vi "Identify Head vs Tail in Difference Image.vi"(8 "significance level":dbl=0.01, 9 "History Length \nfor Head v Tail Determination":i32=100, 10 "Reset?":bool, 11 "Diff Image In":T1) -> (2 "Significant?":bool, 3 "Facing Left?":bool)   [LabVIEW 2011]
uses:
  <vilib>/vision/Image Controls.llb/IMAQ Image.ctl
  <vilib>/Analysis/3filter.llb/Filter Passband Type.ctl
  <vilib>/gmath/statdist.llb/Wilcoxon Signed-Rank Test (mean).vi
  <vilib>/ptbypt/NI_PtbyPt.lvlib
  <vilib>/gmath/NI_Gmath.lvlib
  <vilib>/Analysis/NI_AALBase.lvlib
panel:
  out "Left/Right Diff Sum":i16(graph)
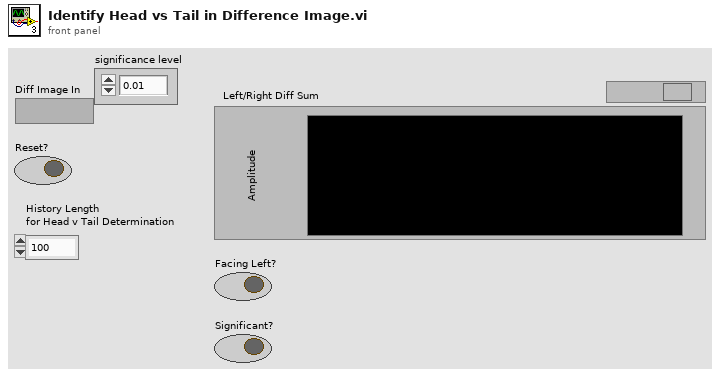
[diagram p1: front panel]
types:
  T1 = typedef "IMAQ Image.ctl" = refnum<image>
  T2 = typedef "NI_AALBase.lvlib/Filter Passband Type.ctl" = enum32{"Lowpass", "Highpass", "Bandpass", "Bandstop"}
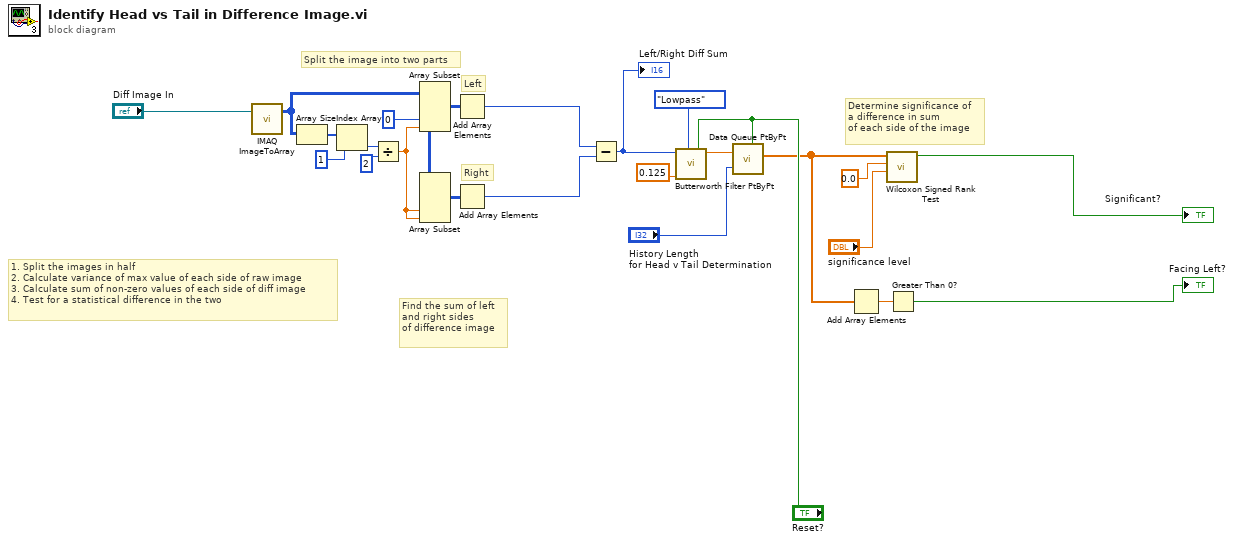
[diagram p0: block diagram]
diagram:
  # "Determine significance of\na difference in sum\nof each side of the image"
  # "Right"
  # "Left"
  # "Split the image into two parts"
  # "Find the sum of left and right sides\nof difference image"
  # "1. Split the images in half\n2. Calculate variance of max value of each side of raw image\n3. Calculate sum of non-zero values of each side of diff image\n4. Test for a statistical difference in the two"
  n1 = call "IMAQ ImageToArray"("Image"="Diff Image In") -> ("Image Pixels (I16)"=w7:i16[][])  [unwired: 3 in, 4 out]
  n2 = Array Size(array=w7) -> (size(s)=w2:i32[])
  n3 = Index Array(array=w2, index=1) -> (element=w4:i32)
  n4 = Divide(x=w4, y=2) -> (x/y=w8:dbl)
  n5 = Array Subset(array=w7, index (col)=0 ("index"), length (col)=w8) -> (w9:i16[][])  [unwired: 2 in]
  n6 = Array Subset(array=w7, index (col)=w8, length (col)=w8) -> (w10:i16[][])  [unwired: 2 in]
  n7 = Add Array Elements(numeric array=w9) -> (sum=w11:i16)
  n8 = Add Array Elements(numeric array=w10) -> (sum=w12:i16)
  n9 = Subtract(x=w11, y=w12) -> (x-y=w18:i16)
  "Left/Right Diff Sum" <- w18
  n10 = call <vilib>:"Butterworth Filter PtByPt.vi"("initialize"="Reset?", "filter type"=Filter_Passband_Type."Lowpass", "low cutoff freq: fl"=0.125, "x"=w18) -> ("Filtered x"=w19:dbl)  [unwired: 5 in, 1 out]
  n11 = call <vilib>:"Data Queue PtByPt.vi"("input data point"=w19, "sample length"="History Length \nfor Head v Tail Determination", "initialize"="Reset?") -> ("Current Queue"=w20:dbl[])  [unwired: 4 out]
  n12 = Add Array Elements(numeric array=w20) -> (sum=w15:dbl)
  n13 = call-poly <vilib>:"Wilcoxon Signed Rank Test.vi"("significance level"="significance level", "mean"=0.0, "sample set"=w20) -> ("reject null hypothesis"=→"Significant?":bool)  [unwired: 6 in, 2 out]
  n14 = Greater Than 0?(x=w15) -> (x > 0?=→"Facing Left?":bool)
